vi "set_ref_clus_MKS670.vi"(6 "input cluster":T1, 10 "pressure":dbl, 11 "status":bool) -> ()   [LabVIEW 2019]
uses:
  cluster_ref_MKS670.ctl
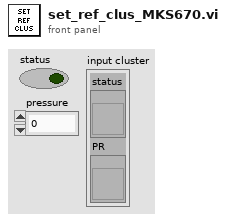
[diagram p1: front panel]
types:
  T1 = typedef "cluster_ref_MKS670.ctl" = cluster{"status":refnum<vi>, "PR":refnum<vi>}
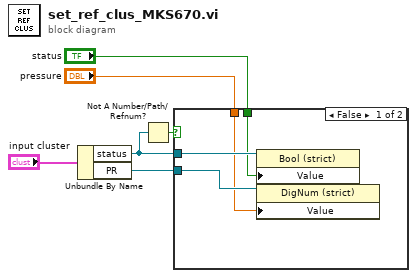
[diagram p0: block diagram]
diagram:
  n1 = Unbundle By Name("input cluster") -> ("status"=w5:refnum<vi>, "PR"=w4:refnum<vi>)
  n2 = Not A Number/Path/Refnum?(number/path/refnum=w5) -> (NaN/Path/Refnum?=w6:bool)
  n3 = case shown="False" w6 {
    tunnel: w5 -> [w10 _]
    tunnel: w4 -> [w9 _]
    tunnel: "status" -> [w8 _]
    tunnel: "pressure" -> [w7 _]
    frame False {
      n4 = property class="Bool (strict)"(reference=w10, "Value"=w8) -> ()  [unwired: 1 in, 2 out]
      n5 = property class="DigNum (strict)"(reference=w9, "Value"=w7) -> ()  [unwired: 1 in, 2 out]
    }
    frame True {
    }
  }
